vi "WPI_UtilitiesFRC FPGATime.vi"(8 "error in (no error)":errorcluster) -> (0 "error out":errorcluster, 3 "FPGA Time":dbl)   [LabVIEW 2025]
doc: "Returns the current time reading of the clock on the FPGA image on the roboRIO device.\n\nThe <b>TimeStamp</b> parameter of the Interrupt Wait VI and the Direct Memory Access (DMA) stream both return the time on the clock.\n\nThis software is licensed. Open the labview\\readme\\WPI Robotics Library Open Source License.txt file for more information."
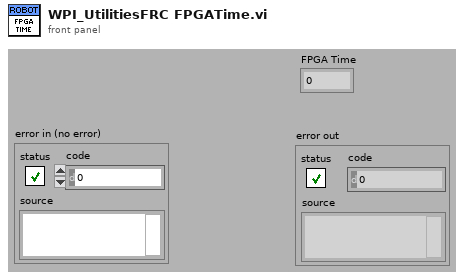
[diagram p1: front panel]
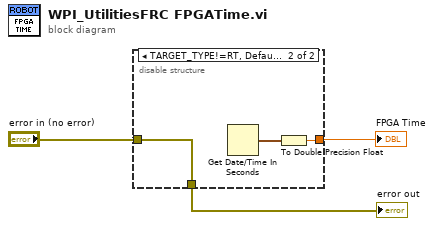
[diagram p0: block diagram]
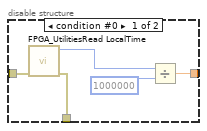
[diagram p2: hidden frame]
diagram:
  n1 = disable-structure shown="TARGET_TYPE!=RT, Default" {
    disable-tunnel: [w6 w11] -> w3
    disable-tunnel: "error in (no error)" -> [w5 w9]
    disable-tunnel: [w4 w9] -> w1
    frame condition #0 {
      n2 = call <vilib>:"FPGA_UtilitiesRead LocalTime.vi"("error in (no error)"=w5) -> ("error out"=w4:errorcluster, "LocalTime"=w8:u32)  [unwired: 9 out]
      n3 = Divide(x=w8, y=u32 1000000) -> (x/y=w6:dbl)
    }
    frame condition #1 (active) {
      n4 = Get Date/Time In Seconds() -> (seconds since 1Jan1904=w10:timestamp)
      n5 = To Double Precision Float(number=w10) -> (double precision float=w11:dbl)
    }
  }
  "FPGA Time" <- w3
  "error out" <- w1
